vi "NI VeriStand - Close Single Waveform Read Session (DBL).vi"(8 "error in (no error)":errorcluster, 11 "Single Waveform Read Session (DBL)":refnum<class "Single Waveform Read (DBL).lvclass">) -> (0 "error out":errorcluster)   [LabVIEW 2020, in "NI_VS Custom Device Waveform API.lvlib" / "Single Waveform Read (DBL).lvclass"]
doc: "Closes a waveform read or write session. Wire data to the <B>Single Waveform Read Session (DBL)</B> input to specify the instance to use."
uses:
  Single Waveform Read (DBL).lvclass
  D:/p4/penguin/lvaddon/Veristand/master/src/LabVIEW/vilib/NI VeriStand/Custom Device Waveform API/Waveform Session.lvclass
  Waveform Session.lvclass/Waveform Session.ctl
  Single Waveform Read (DBL).lvclass/Single Waveform Read (DBL).ctl
  Internal Comm Classes/WPL Comm/WPL Comm.lvclass/WPL Comm.ctl
  Internal Comm Classes/WPL Comm/WPL Comm (1D DBL)/WPL Comm (1D DBL).lvclass/WPL Comm (1D DBL).ctl
  Internal Comm Classes/WPL Comm/Read Access.vi
  Internal Comm Classes/WPL Comm/WPL Comm (1D DBL)/Set 1D DBL Read Q on Variant.vi
  Internal Comm Classes/WPL Comm/WPL_close waveform.vi
  Internal Comm Classes/WPL Comm/Convert Q Error to Shutdown Error.vi
  Internal Comm Classes/WPL Comm/Set ErrorQ on Variant.vi
  Internal Comm Classes/WPL Comm/Send WPL Command.vi
  Internal Comm Classes/WPL Comm/WPL Comm (1D DBL)/WPL Comm (1D DBL).lvclass
  D:/p4/penguin/lvaddon/Veristand/master/src/LabVIEW/vilib/NI VeriStand/Custom Device Waveform API/Internal Comm Classes/WPL Comm/WPL Comm.lvclass
  <vilib>/Utility/error.llb/Error Cluster From Error Code.vi
  Waveform Session.lvclass
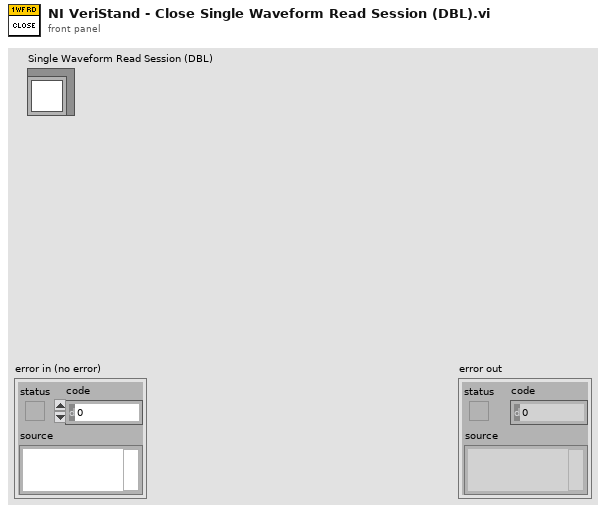
[diagram p1: front panel]
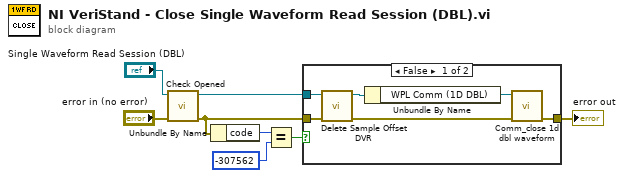
[diagram p0: block diagram]
diagram:
  n1 = call "Check Opened.vi"("error in (no error)"="error in (no error)", "Waveform Session in"="Single Waveform Read Session (DBL)") -> ("error out"=w4:errorcluster, "Waveform Session out"=w5:refnum<class "Single Waveform Read (DBL).lvclass">)  [unwired: 8 in]
  n2 = Unbundle By Name(w4) -> ("code"=w2:i32)
  n3 = Equal?(x=w2, y=-307562 ("error code (0)")) -> (x = y?=w1:bool)
  n4 = case shown="False" w1 {
    tunnel: [w14 w15] -> w7
    tunnel: w5 -> [w13 _]
    tunnel: w4 -> [w9 w15]
    frame False {
      n5 = call "Delete Sample Offset DVR.vi"("error in (no error)"=w9, "Waveform Session in"=w13) -> ("error out"=w10:errorcluster, "Waveform Session out"=w12:refnum<class "Single Waveform Read (DBL).lvclass">)  [unwired: 8 in]
      n6 = Unbundle By Name(w12) -> ("WPL Comm (1D DBL)"=w11:refnum<class "WPL Comm (1D DBL).lvclass">)
      n7 = call "Comm_close 1d dbl waveform.vi"("error in (no error)"=w10, "WPL Comm (1D DBL) in"=w11) -> ("error out"=w14:errorcluster)  [unwired: 9 in]
    }
    frame True {
    }
  }
  "error out" <- w7
